vi "send power.vi"(5 "packet start":bool, 9 "input valid":bool, 10 "sample":T1) -> ()   [LabVIEW 2020]
uses:
  <vilib>/rvi/interface/RandomDataEmulation/niFpgaRandomDataHandleErrors.vi
  <vilib>/rvi/DataTransferAndStorage/Container/XNode/niFpgaContainer.xnode
  <vilib>/rvi/interface/RandomDataEmulation/nirviRandomDataFpgaReadWriteTemplate.vi
types:
  T1 = cluster{"Real":fxp<+/-,16,3>, "Imag":fxp<+/-,16,3>}
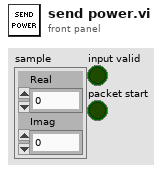
[diagram p1: front panel]
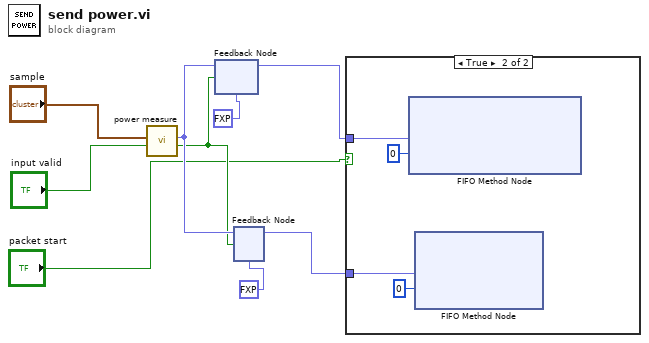
[diagram p0: block diagram]
diagram:
  n1 = call "power measure.vi"("input valid"="input valid", "sample"="sample") -> ("output valid"=w4:bool, "output"=w6:fxp<+,38,6>)  [unwired: 8 in]
  n2 = feedback-in #1(w6, w4) -> ()
  n3 = feedback #1(fxp<+,38,6> 0.0 ("output")) -> (w7:fxp<+,38,6>)
  n4 = feedback #2(fxp<+,38,6> 0.0 ("output")) -> (w5:fxp<+,38,6>)
  n5 = feedback-in #2(w6, w4) -> ()
  n6 = case shown="True" "packet start" {
    tunnel: w7 -> [_ w13]
    tunnel: w5 -> [_ w12]
    frame False {
    }
    frame True {
      n7 = xnode ("FIFO Method Node")("Element"=w13, "Timeout"=0) -> ()  [unwired: 1 in, 2 out]
      n8 = xnode ("FIFO Method Node")("Element"=w12, "Timeout"=0) -> ()  [unwired: 1 in, 2 out]
    }
  }
